vi "RIO Fusion Multicast Receiver.vi"() -> ()   [LabVIEW 2015]
doc: "Creates a read-only UDP multicast session and receives data on the specified port."
uses:
  <vilib>/Utility/tcp.llb/UDP Multicast Read-Only Open.vi
panel:
  out "address":u32
  out "port":u16
  out "Sensor Fusion Data":dbl(graph)
  in  "Stop":bool
  # "Overview: Demonstrates the use of the UDP functions to connect to a UDP multicast session and receive data.\nInstructions:\n1. Ensure UDP Multicast - Sender.vi is already running.\n2. Run the VI.\n3. Click Stop to stop the VI."
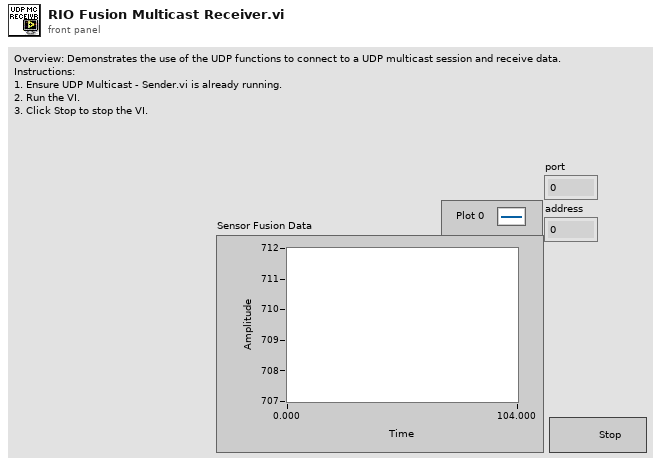
[diagram p1: front panel]
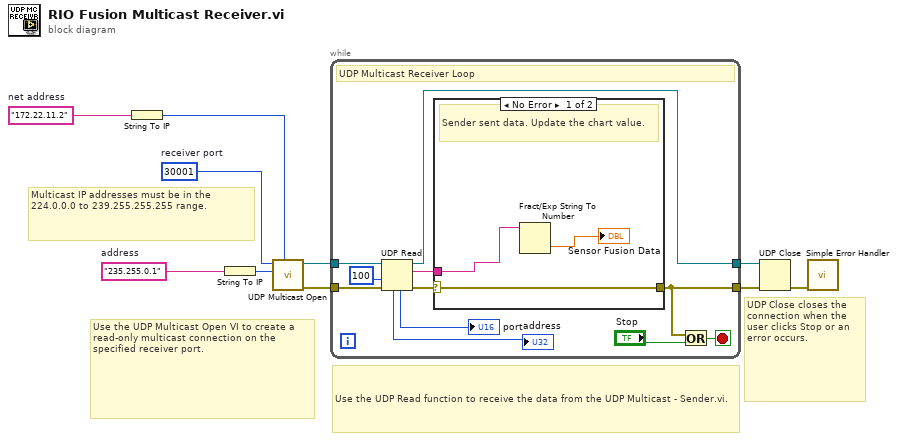
[diagram p0: block diagram]
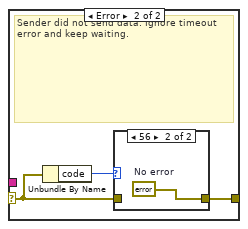
[diagram p2: hidden frame]
diagram:
  w1 = "172.22.11.2"  # net address
  w4 = u16 30001  # receiver port
  w9 = "235.255.0.1"  # address
  # "UDP Close closes the connection when the user clicks Stop or an error occurs."
  # "Use the UDP Multicast Open VI to create a read-only multicast connection on the specified receiver port."
  # "Multicast IP addresses must be in the 224.0.0.0 to 239.255.255.255 range."
  # "Use the UDP Read function to receive the data from the UDP Multicast - Sender.vi."
  n1 = String To IP(1:w1) -> (0:w2:u32)
  n2 = String To IP(1:w9) -> (0:w3:u32)
  n3 = call-poly <vilib>:"UDP Multicast Open.vi"("net address"=w2, "multicast addr"=w3, "port"=w4) -> ("error out"=w6:errorcluster, "connection ID"=w5:refnum<k16>)  [unwired: 6 in, 1 out]
  n4 = while {
    tunnel: w5 -> [w21]
    tunnel: [w13] -> w10
    tunnel: w6 -> [w18]
    tunnel: [w14] -> w7
    stop <- w19 stop-if-true
    # "UDP Multicast Receiver Loop"
    n5 = UDP Read(connection ID=w21, timeout ms (25000)=100, 8:w18) -> (data out=w16:string, error out=w15:errorcluster, 3:w13:refnum<k16>, 4:→"port":u16, 6:→"address":u32)  [unwired: 1 out]
    n6 = case shown="No Error" w15 {
      selector: w15 -> [w24 w26]
      tunnel: w16 -> [w23 _]
      tunnel: [w24 w25] -> w14
      frame No Error {
        # "Sender sent data. Update the chart value."
        n7 = Fract/Exp String To Number(string=w23) -> (number=→"Sensor Fusion Data":dbl)  [unwired: 3 in, 1 out]
      }
      frame Error {
        # "Sender did not send data. Ignore timeout error and keep waiting."
        n8 = Unbundle By Name(w26) -> ("code"=w27:i32)
        n9 = case shown="56" w27 {
          tunnel: w26 -> [w28 _]
          tunnel: [w28 w29] -> w25
          frame Default {
          }
          frame 56 {
            w29 = errorcluster {"status"=FALSE, "code"=0, "source"=""}  # No error
          }
        }
      }
    }
    n10 = Or(x=w14, y="Stop") -> (x .or. y?=w19:bool)
  }
  n11 = UDP Close(connection ID=w10, 8:w7) -> (error out=w8:errorcluster)  [unwired: 1 out]
  n12 = call <vilib>:"Simple Error Handler.vi"("error in (no error)"=w8) -> ()  [unwired: 1 in, 8 out]
